vi "RoiLoopAndorNull.vi"(3 "queue in":refnum<queue>, 11 "error in":errorcluster) -> (6 "ROI Intensity Graph Out":i32[][](graph), 15 "error out 2":errorcluster)   [LabVIEW 2011]
panel:
  in  "OldDatain":i32[][](array[numeric])
  in  "Array 2":i32[][][](array[numeric])
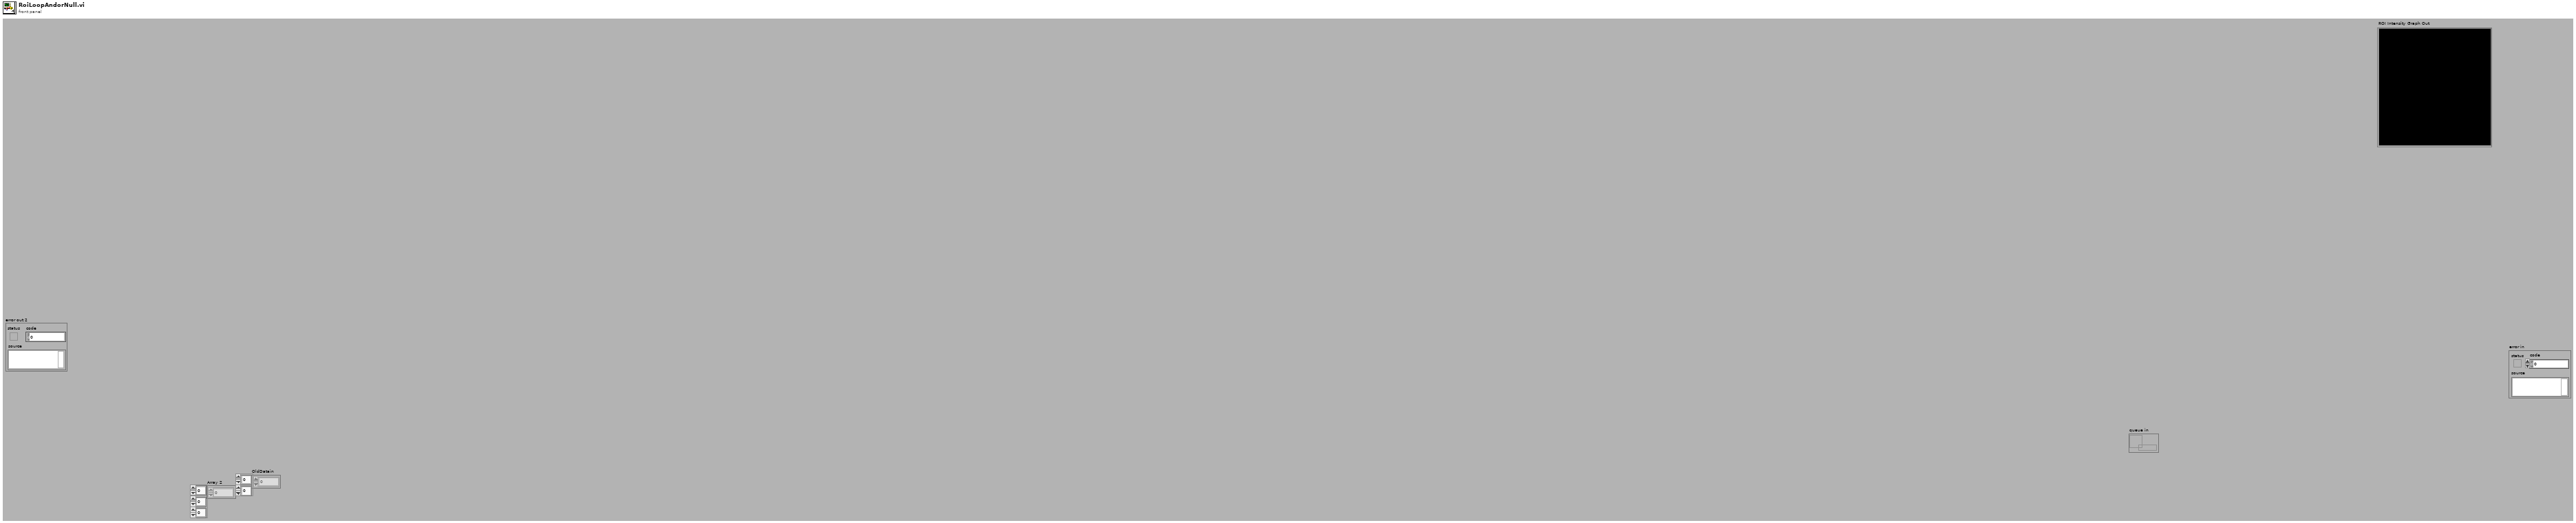
[diagram p1: front panel]
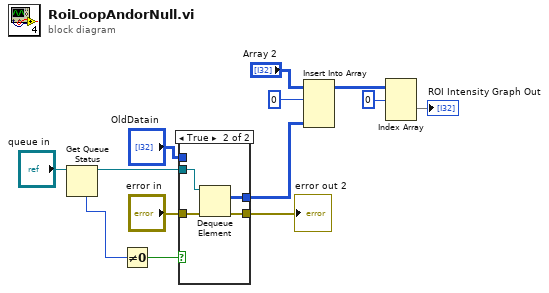
[diagram p0: block diagram]
diagram:
  n1 = Get Queue Status(queue="queue in") -> (queue out=w1:refnum<queue>, # elements in queue=w3:i32)  [unwired: 2 in, 6 out]
  n2 = Not Equal To 0?(x=w3) -> (x != 0?=w12:bool)
  n3 = case shown="True" w12 {
    tunnel: "error in" -> [w15 w19]
    tunnel: [w15 w17] -> w6
    tunnel: w1 -> [_ w18]
    tunnel: [w14 w16] -> w7
    tunnel: "OldDatain" -> [w14 _]
    frame False {
    }
    frame True {
      n4 = Dequeue Element(queue=w18, error in (no error)=w19) -> (element=w16:i32[][], error out=w17:errorcluster)  [unwired: 1 in, 2 out]
    }
  }
  "error out 2" <- w6
  n5 = Insert Into Array(array="Array 2", index (dim 0)=0 ("index (page)"), new element=w7) -> (w10:i32[][][])  [unwired: 2 in]
  n6 = Index Array(array=w10, index (dim 0)=0 ("index (page)")) -> (element=→"ROI Intensity Graph Out":i32[][])  [unwired: 2 in]
